vi "get TGA_DSC queue.vi"(8 "error in":errorcluster, 10 "statusRef":refnum<vi>, 11 "queue in":refnum<queue>) -> (0 "错误输出 2":errorcluster caption="error out", 3 "queue out":refnum<queue>)   [LabVIEW 2011]
uses:
  dataType/TGA_DSC new data record.ctl
  dataType/TGA_DSC.ctl
panel:
  in  "DBSet":T1={"Server"="172.20.23.107", "DB"="MESDATACenter", "PSW"="data'songyy", "User"="sa"}
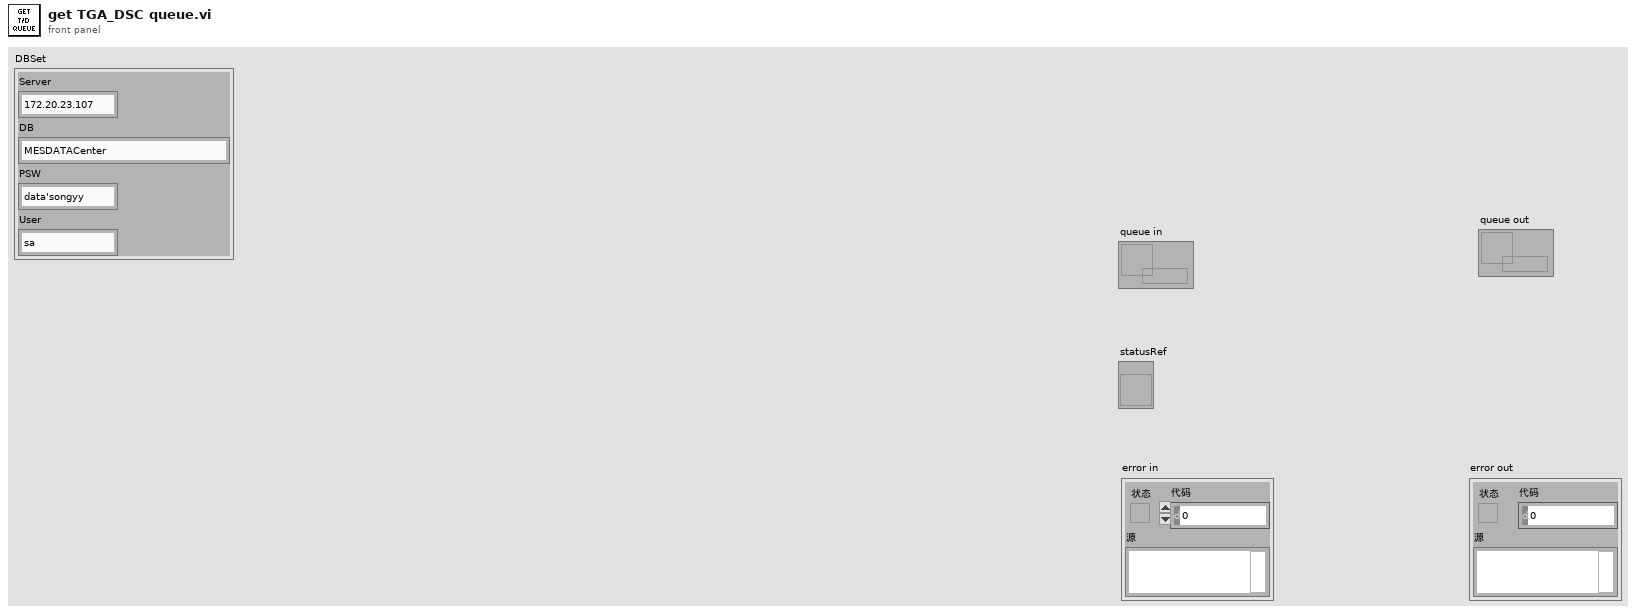
[diagram p1: front panel]
types:
  T1 = cluster{"Server":string, "DB":string, "PSW":string, "User":string}
  T2 = typedef "TGA_DSC new data record.ctl" = cluster{"id":string, "TGA/DSC":T3, "txtPath":path, "num":dbl, "lastone?":bool}
  T3 = typedef "TGA_DSC.ctl" = cluster{"materialCode":string, "SN":string, "pcName":string, "programmName":string, "startTime":string, "stopTime":string, "itemName":string}
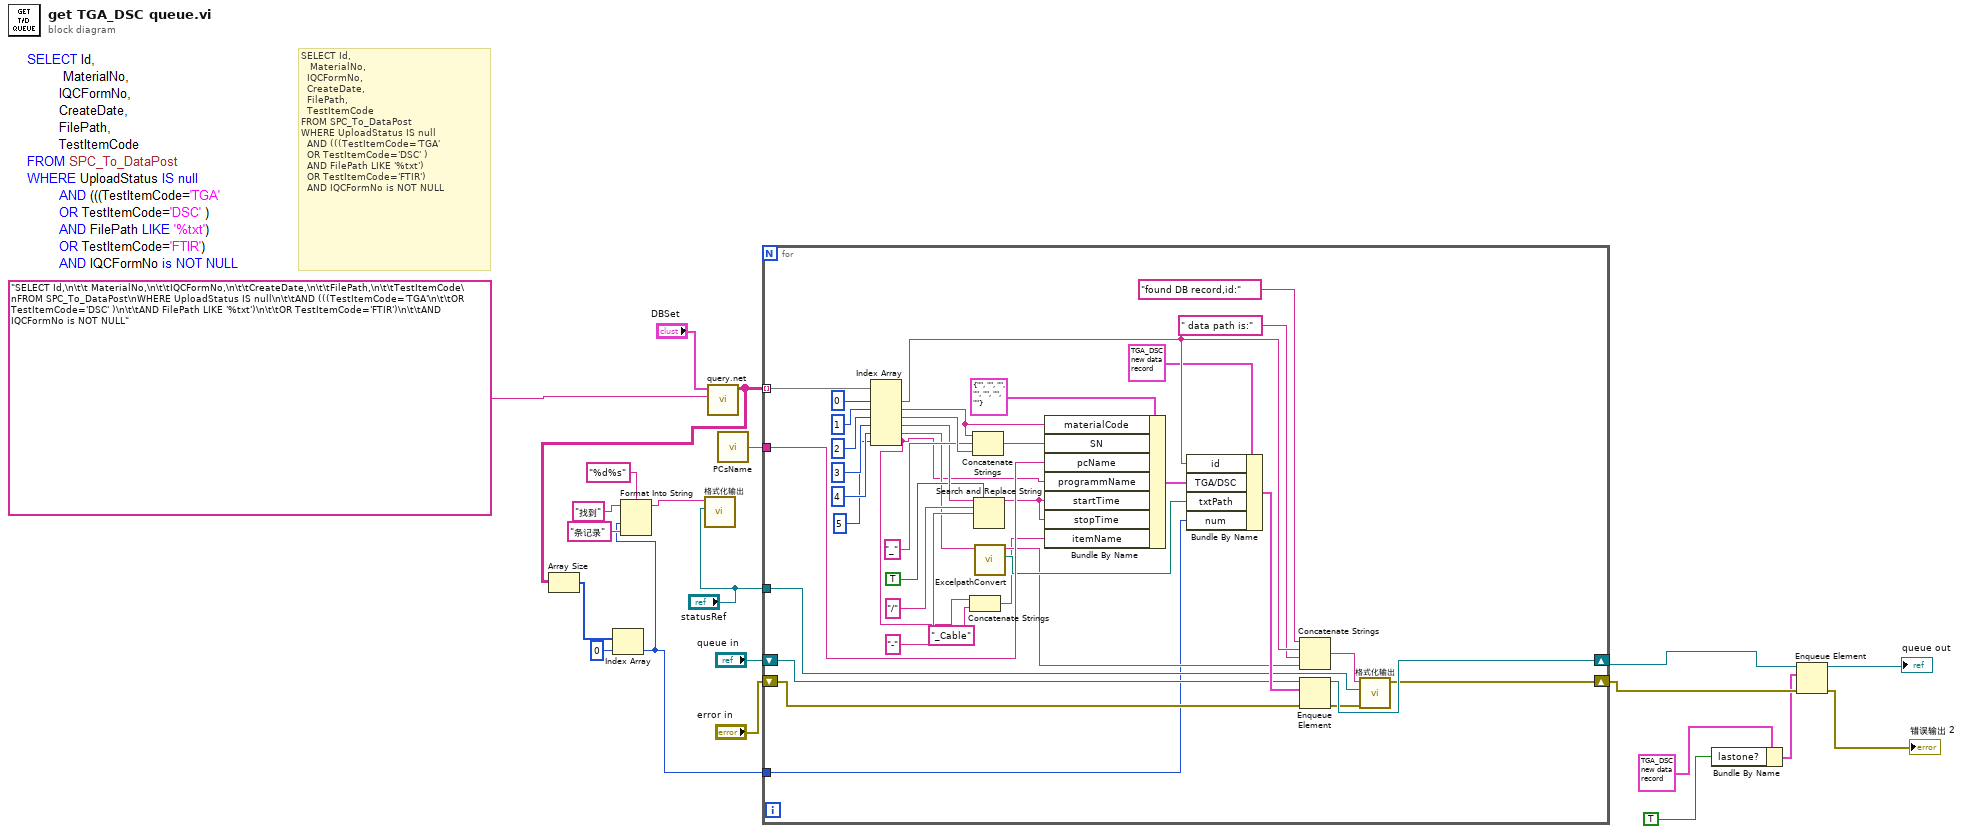
[diagram p0: block diagram]
diagram:
  # "SELECT Id,\n\t\t MaterialNo,\n\t\tIQCFormNo,\n\t\tCreateDate,\n\t\tFilePath,\n\t\tTestItemCode\nFROM SPC_To_DataPost\nWHERE UploadStatus IS null\n\t\tAND (((TestItemCode='TGA'\n\t\tOR TestItemCode='DSC' )\n\t\tAND FilePath LIKE '%txt')\n\t\tOR TestItemCode='FTIR')\n\t\tAND IQCFormNo is NOT NULL"
  n1 = call "query.net.vi"("Sql"="SELECT Id,\n\t\t MaterialNo,\n\t\tIQCFormNo,\n\t\tCreateDate,\n\t\tFilePath,\n\t\tTestItemCode\nFROM SPC_To_DataPost\nWHERE UploadStatus IS null\n\t\tAND (((TestItemCode='TGA'\n\t\tOR TestItemCode='DSC' )\n\t\tAND FilePath LIKE '%txt')\n\t\tOR TestItemCode='FTIR')\n\t\tAND IQCFormNo is NOT NULL", "DBSet"="DBSet") -> ("result"=w16:string[][])  [unwired: 8 in, 1 out]
  n2 = Array Size(array=w16) -> (size(s)=w15:i32[])
  n3 = Index Array(array=w15, index=0 ("索引")) -> (element=w1:i32)
  n4 = Format Into String(format string="%d%s" ("格式字符串"), initial string="找到" ("输入字符串"), w1, "条记录" ("输入 2")) -> (resulting string=w2:string)  [unwired: 1 in, 1 out]
  n5 = call "格式化输出.vi"("字符串引用"="statusRef", "字符串"=w2) -> ()  [unwired: 9 in, 1 out]
  n6 = call "PCsName.vi"() -> ("Computer Name"=w19:string)
  n7 = for {
    tunnel: w16 -> [w58] mode=indexing
    tunnel: w19 -> [w51]
    shift-right: [w37] -> w13
    shift-left: "queue in" -> [w38]
    tunnel: "statusRef" -> [w36]
    shift-right: [w29] -> w11
    shift-left: "error in" -> [w28]
    tunnel: w1 -> [w27]
    n8 = Index Array(array=w58, index #1=0 ("索引"), index #2=1 ("索引"), index #3=2 ("索引"), index #4=3 ("索引"), index #5=4 ("索引"), index #6=5 ("索引")) -> (element #1=w34:string, element #2=w55:string, element #3=w54:string, element #4=w49:string, element #5=w42:string, element #6=w25:string)
    n9 = Concatenate Strings(w25, "_Cable" ("字符串")) -> (w24:string)
    n10 = Concatenate Strings(w55, "_" ("字符串"), w54) -> (w53:string)
    n11 = Search and Replace String(replace all?=TRUE ("替换全部？(F)"), input string=w49, search string="/" ("搜索字符串"), replace string="-" ("替换字符串(\"\")")) -> (result string=w45:string)  [unwired: 4 in, 3 out]
    n12 = call "ExcelpathConvert.vi"("输入字符串"=w42) -> ("路径"=w40:path, "结果字符串"=w32:string)  [unwired: 9 in]
    n13 = Bundle By Name(cluster=T3 {"materialCode"="", "SN"="", "pcName"="", "programmName"="", "startTime"="", "stopTime"="", "itemName"=""} ("簇"), "materialCode"=w55, "SN"=w53, "pcName"=w51, "programmName"=w25, "startTime"=w45, "stopTime"=w45, "itemName"=w24) -> (w41:T3)
    n14 = Bundle By Name(cluster=T2 {"id"="", "TGA/DSC"={"materialCode"="", "SN"="", "pcName"="", "programmName"="", "startTime"="", "stopTime"="", "itemName"=""}, "txtPath"=path "", "num"=0.0, "lastone?"=FALSE} ("TGA/DSC new data"), "id"=w34, "TGA/DSC"=w41, "txtPath"=w40, "num"=w27) -> (w39:T2)
    n15 = Concatenate Strings("found DB record,id:", w34, " data path is:" ("字符串"), w32) -> (w31:string)
    n16 = Enqueue Element(queue=w38, element=w39, error in (no error)=w28) -> (queue out=w37:refnum<queue>, error out=w30:errorcluster)  [unwired: 1 in, 1 out]
    n17 = call "格式化输出.vi"("错误输入（无错误）"=w30, "字符串引用"=w36, "字符串"=w31) -> ("错误输出"=w29:errorcluster)  [unwired: 8 in]
  }
  n18 = Bundle By Name(cluster=T2 {"id"="", "TGA/DSC"={"materialCode"="", "SN"="", "pcName"="", "programmName"="", "startTime"="", "stopTime"="", "itemName"=""}, "txtPath"=path "", "num"=0.0, "lastone?"=FALSE} ("TGA/DSC new data"), "lastone?"=TRUE) -> (w8:T2)
  n19 = Enqueue Element(queue=w13, element=w8, error in (no error)=w11) -> (queue out=→"queue out":refnum<queue>, error out=→"错误输出 2":errorcluster)  [unwired: 1 in, 1 out]
